vi "Test Plugins.vi"(8 "Error In":errorcluster, 10 "Plugin Data":T1, 11 "Factory Plugin Framework in":refnum<class "Factory Plugin Framework.lvclass">=refnum) -> (0 "Error Out":errorcluster, 3 "Factory Plugin Framework out":refnum<class "Factory Plugin Framework.lvclass">)   [LabVIEW 2018, in "Factory Plugin Framework.lvlib" / "Factory Plugin Framework.lvclass"]
uses:
  Factory Plugin Framework.lvclass
  Factory Plugin Framework.lvclass/Factory Plugin Framework.ctl
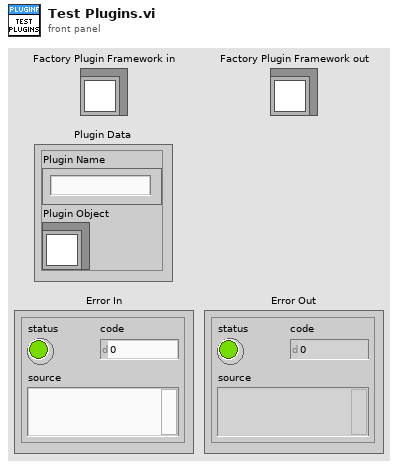
[diagram p1: front panel]
types:
  T1 = cluster{"Plugin Name":string, "Plugin Object":refnum<class>}
  T2 = cluster{"Plugin Name":string, "Plugin Object":refnum<class>}[]
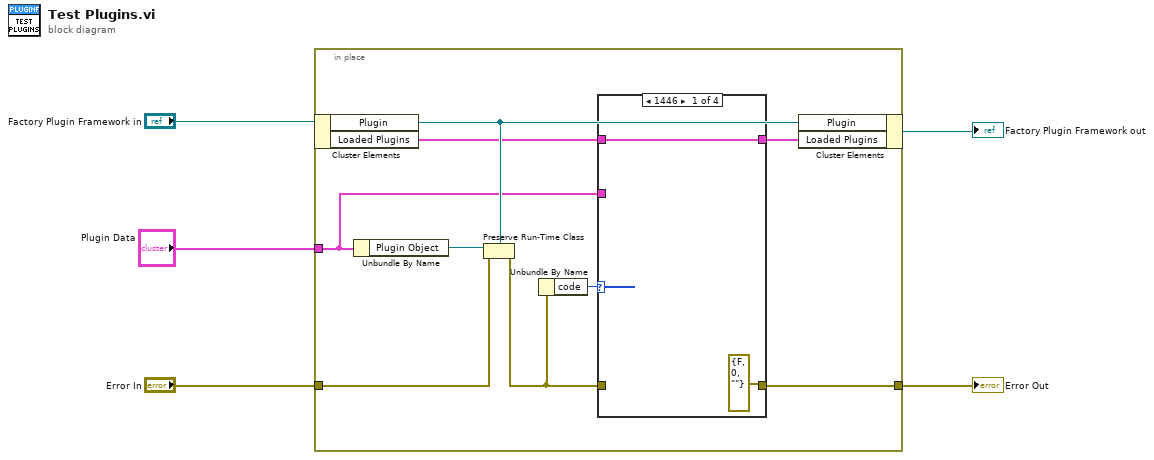
[diagram p0: block diagram]
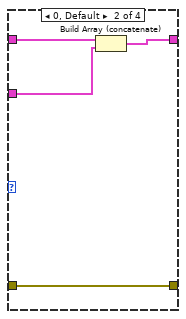
[diagram p2: hidden frame]
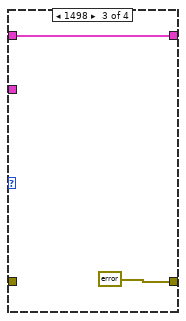
[diagram p3: hidden frame]
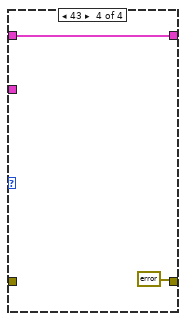
[diagram p4: hidden frame]
diagram:
  n1 = in-place {
    in-place-border: [w14] -> w5
    in-place-border: "Error In" -> [w11]
    in-place-border: "Plugin Data" -> [w7]
    n2 = in-place-cluster #1("Factory Plugin Framework in") -> ("Plugin"=w10:refnum<class>, "Loaded Plugins"=w9:T2)
    n3 = Unbundle By Name(w7) -> ("Plugin Object"=w8:refnum<class>)
    n4 = Preserve Run-Time Class(object in=w8, error in=w11, 2:w10) -> (error out=w12:errorcluster)  [unwired: 1 out]
    n5 = Unbundle By Name(w12) -> ("code"=w13:i32)
    n6 = case shown="1446" w13 {
      tunnel: [errorcluster {"status"=FALSE, "code"=0, "source"=""} ("error constant") w19 errorcluster {"status"=FALSE, "code"=0, "source"=""} ("error constant") errorcluster {"status"=FALSE, "code"=0, "source"=""} ("error constant")] -> w14
      tunnel: w12 -> [_ w19 _ _]
      tunnel: w9 -> [w15 w20 w21 w23]
      tunnel: [w15 w18 w21 w23] -> w6
      tunnel: w7 -> [_ w17 _ _]
      frame 1446 {
      }
      frame 0, Default {
        n7 = Build Array (concatenate)(w20, w17) -> (w18:T2)
      }
      frame 1498 {
      }
      frame 43 {
      }
    }
    n8 = in-place-cluster #1("Plugin"=w10, "Loaded Plugins"=w6) -> (→"Factory Plugin Framework out":refnum<class "Factory Plugin Framework.lvclass">)
  }
  "Error Out" <- w5
